vi "Get Broken VI Key Names.vi"() -> (2 "Before Build Key":string, 3 "Broken VIs List Key":string)   [LabVIEW 2020, in "AB_Build.lvclass"]
uses:
  <vilib>/AppBuilder/AB_Classes/Build/AB_Build.lvclass
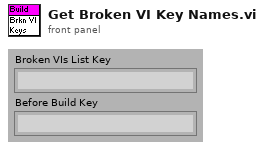
[diagram p1: front panel]
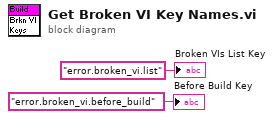
[diagram p0: block diagram]
diagram:
  "Broken VIs List Key" <- "error.broken_vi.list" ("y")
  "Before Build Key" <- "error.broken_vi.before_build" ("Key")
